vi "Display.vi"(0 "Data In":T4 {"time" format="%<%H:%M:%S%2u>T"}, 2 "Display State In":T2, 3 "Container State":T3) -> (6 "Data Out":T4 {"time" format="%<%H:%M:%S%2u>T"}, 7 "Display State Out":T2, 8 "Action":T1)   [LabVIEW 2015, in "Configurable Buffer.xctl"]
uses:
  Configurable Buffer.xctl
  Data.ctl
  <vilib>/_xctls/Container State.ctl
  State.ctl
  <vilib>/_xctls/Action.ctl
  <vilib>/_xctls/XControlSupport.lvlib
panel:
  out "plot":cluster{"Time":timestamp[], dbl[]}[](graph)
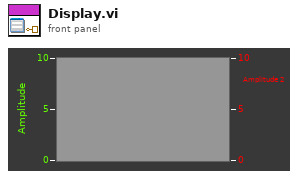
[diagram p1: front panel]
types:
  T1 = typedef "XControlSupport.lvlib/Action.ctl" = cluster{"Data Changed?":bool, "State Changed?":bool, "Action Name":string}
  T2 = typedef "Configurable Buffer.xctl/State.ctl" = cluster{"Plot Ref":refnum<vi>, "History":i32}
  T3 = typedef "XControlSupport.lvlib/Container State.ctl" = cluster{"Indicator?":bool, "Run Mode?":bool, " Refnum":refnum<vi>}
  T4 = typedef "Configurable Buffer.xctl/Data.ctl" = cluster{"Val":dbl[], "time":timestamp}
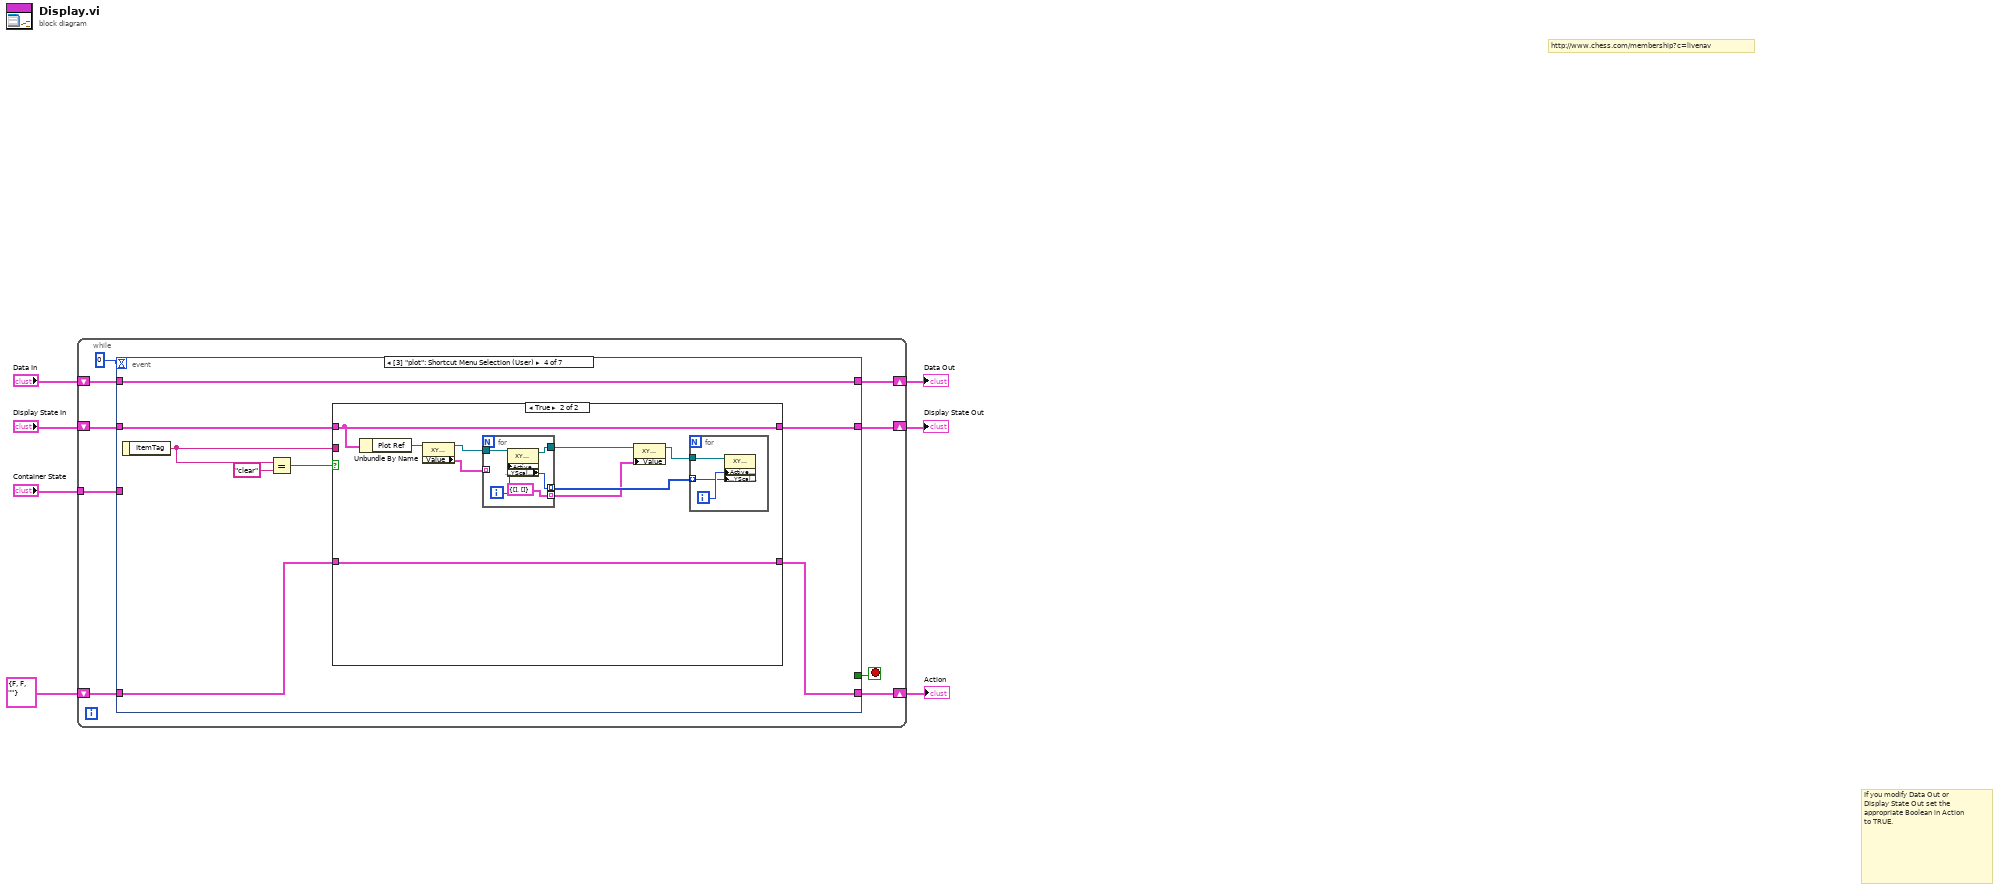
[diagram p0: block diagram]
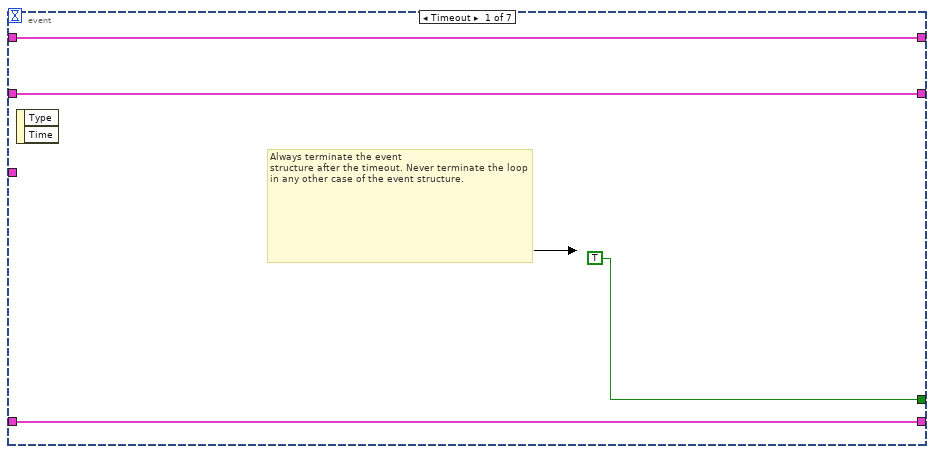
[diagram p2: hidden frame]
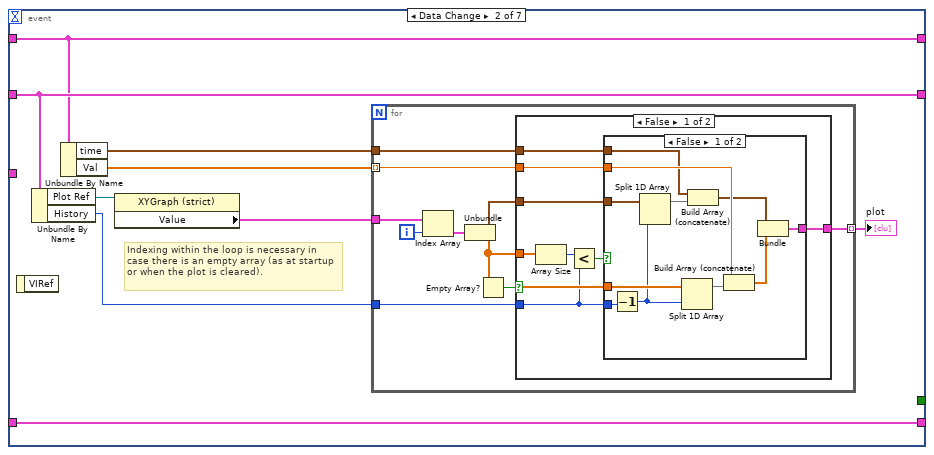
[diagram p3: hidden frame]
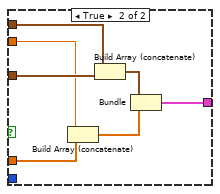
[diagram p4: hidden frame]
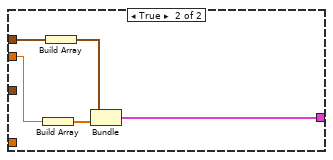
[diagram p5: hidden frame]
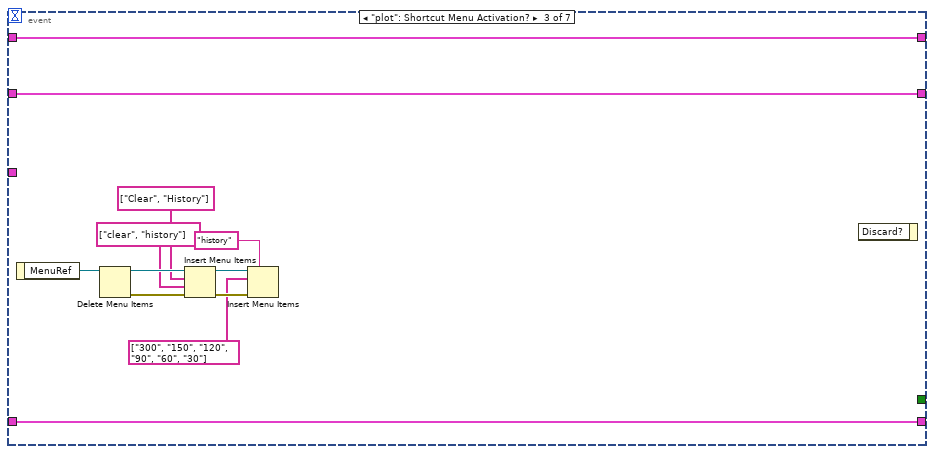
[diagram p6: hidden frame]
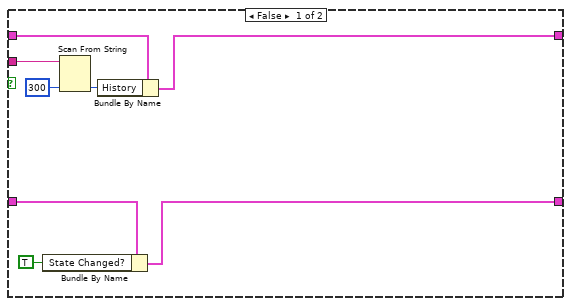
[diagram p7: hidden frame]
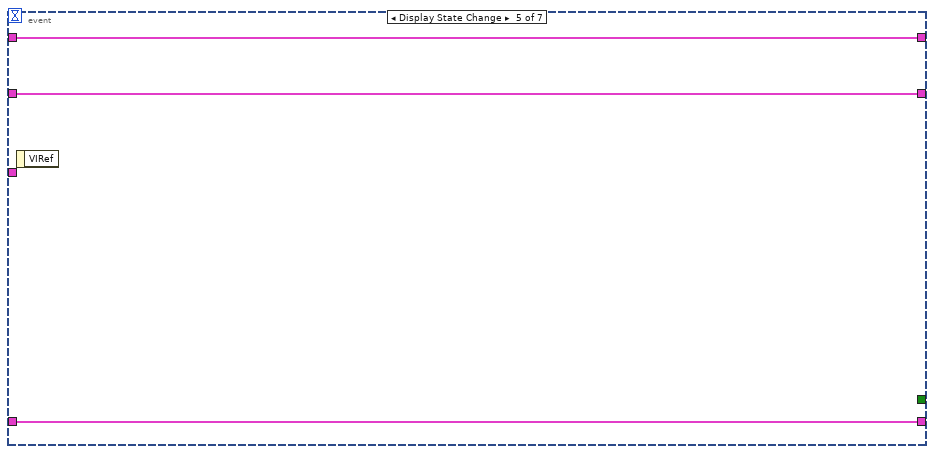
[diagram p8: hidden frame]
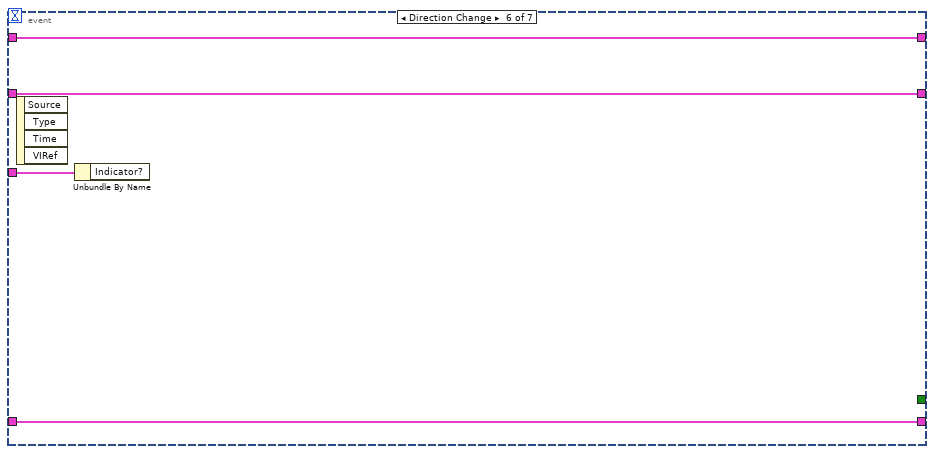
[diagram p9: hidden frame]
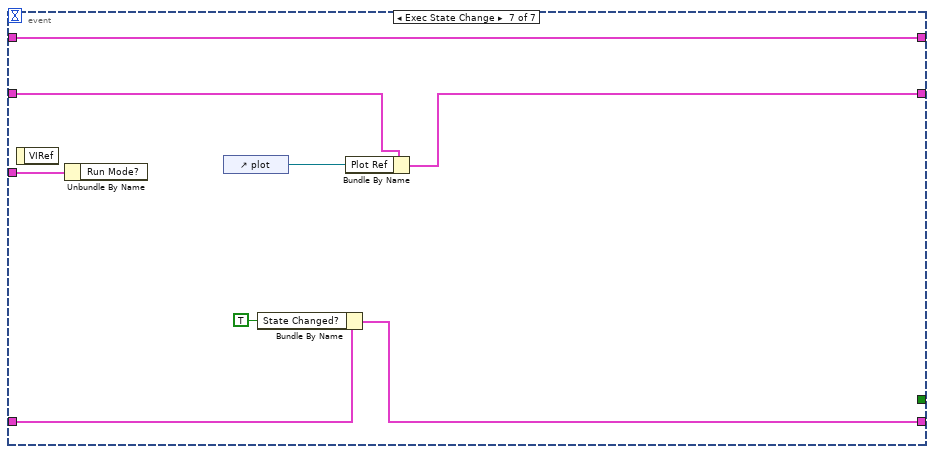
[diagram p10: hidden frame]
diagram:
  # "http://www.chess.com/membership?c=livenav"
  # "If you modify Data Out or\nDisplay State Out set the\nappropriate Boolean in Action\nto TRUE."
  n1 = while {
    shift-right: [w15] -> w4
    shift-left: "Display State In" -> [w16]
    tunnel: "Container State" -> [w12]
    shift-right: [w10] -> w7
    shift-left: "Data In" -> [w11]
    shift-right: [w8] -> w2
    shift-left: T1 {"Data Changed?"=FALSE, "State Changed?"=FALSE, "Action Name"=""} ("Action") -> [w9]
    stop <- w14 stop-if-true
    n2 = event shown="[3] \"plot\": Shortcut Menu Selection (User)" {
      selector: _ -> [_ _ _ _ _ _ _]
      dyn-events: _ -> [_ _ _ _ _ _ _]
      timeout: 0 -> [_ _ _ _ _ _ _]
      tunnel: w16 -> [w18 w29 w82 w86 w118 w121 w128]
      tunnel: [w18 w29 w82 w85 w118 w121 w127] -> w15
      tunnel: [TRUE _ _ _ _ _ _] -> w14
      tunnel: w12 -> [_ _ _ _ _ w122 w130]
      tunnel: w11 -> [w17 w28 w81 w90 w117 w120 w129]
      tunnel: [w17 w28 w81 w90 w117 w120 w129] -> w10
      tunnel: [w19 w27 w80 w83 w116 w119 w125] -> w8
      tunnel: w9 -> [w19 w27 w80 w84 w116 w119 w126]
      event Timeout {
        # "Always terminate the event\nstructure after the timeout. Never terminate the loop in any other case of the event structure."
        n3 = event-data() -> ()  [unwired: 1 in, 2 out]
      }
      event Data Change {
        # "Indexing within the loop is necessary in case there is an empty array (as at startup or when the plot is cleared)."
        n4 = event-data() -> ()  [unwired: 1 in, 1 out]
        n5 = Unbundle By Name(w29) -> ("Plot Ref"=w26:refnum<vi>, "History"=w21:i32)
        n6 = Unbundle By Name(w28) -> ("time"=w24:timestamp, "Val"=w23:dbl[])
        n7 = property on="Property Node" class="XYGraph (strict)"(reference=w26) -> ("Value"=w25:cluster{"Time":timestamp[], dbl[]}[])  [unwired: 1 in, 2 out]
        n8 = for {
          tunnel: w25 -> [w33]
          tunnel: w24 -> [w38]
          tunnel: w23 -> [w37] mode=indexing
          tunnel: [w36] -> w22 mode=indexing
          tunnel: w21 -> [w30]
          i -> [w31]
          n9 = Index Array(array=w33, index=w31) -> (element=w32:cluster{"Time":timestamp[], dbl[]})
          n10 = Unbundle(w32) -> ("Time"=w39:timestamp[], w35:dbl[])
          n11 = Empty Array?(array=w35) -> (empty?=w34:bool)
          n12 = case shown="False" w34 {
            tunnel: w39 -> [w45 _]
            tunnel: w38 -> [w44 w70]
            tunnel: w37 -> [w43 w69]
            tunnel: [w42 w66] -> w36
            tunnel: w35 -> [w41 _]
            tunnel: w30 -> [w40 _]
            frame False {
              n13 = Array Size(array=w41) -> (size(s)=w47:i32)
              n14 = Less?(x=w47, y=w40) -> (x < y?=w46:bool)
              n15 = case shown="False" w46 {
                tunnel: w41 -> [w57 w63]
                tunnel: w45 -> [w58 w64]
                tunnel: w44 -> [w53 w65]
                tunnel: w43 -> [w55 w62]
                tunnel: [w50 w59] -> w42
                tunnel: w40 -> [w49 _]
                frame False {
                  n16 = Decrement(x=w49) -> (x-1=w48:i32)
                  n17 = Split 1D Array(array=w58, index=w48) -> (first subarray=w54:timestamp[])  [unwired: 1 out]
                  n18 = Split 1D Array(array=w57, index=w48) -> (first subarray=w56:dbl[])  [unwired: 1 out]
                  n19 = Build Array (concatenate)(w53, w54) -> (w52:timestamp[])
                  n20 = Build Array (concatenate)(w55, w56) -> (w51:dbl[])
                  n21 = Bundle(w52, w51) -> (w50:cluster{timestamp[], dbl[]})  [unwired: 1 in]
                }
                frame True {
                  n22 = Build Array (concatenate)(w62, w63) -> (w60:dbl[])
                  n23 = Build Array (concatenate)(w65, w64) -> (w61:timestamp[])
                  n24 = Bundle(w61, w60) -> (w59:cluster{timestamp[], dbl[]})  [unwired: 1 in]
                }
              }
            }
            frame True {
              n25 = Build Array(w69) -> (w67:dbl[])
              n26 = Build Array(w70) -> (w68:timestamp[])
              n27 = Bundle(w68, w67) -> (w66:cluster{timestamp[], dbl[]})  [unwired: 1 in]
            }
          }
        }
        "plot" <- w22
      }
      event "plot": Shortcut Menu Activation? {
        n28 = event-data() -> ("MenuRef"=w79:refnum<k9>)  [unwired: 1 in]
        n29 = Delete Menu Items(9:w79) -> (0:w77:errorcluster, 3:w78:refnum<k9>)  [unwired: 3 in]
        n30 = Insert Menu Items(6:w77, 7:string[] ["clear", "history"] ("item tags"), 8:string[] ["Clear", "History"] ("item names"), 9:w78) -> (0:w73:errorcluster, 3:w74:refnum<k9>)  [unwired: 2 in, 1 out]
        n31 = Insert Menu Items(5:"history" ("menu tag"), 6:w73, 8:string[] ["300", "150", "120", "90", "60", "30"] ("item names"), 9:w74) -> ()  [unwired: 2 in, 3 out]
        n32 = event-data() -> ()  [unwired: 2 in, 1 out]
      }
      event "plot": Shortcut Menu Selection (User) {
        n33 = event-data() -> ("ItemTag"=w87:string)  [unwired: 1 in]
        n34 = Equal?(x=w87, y="clear") -> (x = y?=w88:bool)
        n35 = case shown="True" w88 {
          tunnel: w86 -> [w96 w107]
          tunnel: [w94 w107] -> w85
          tunnel: w87 -> [w98 _]
          tunnel: w84 -> [w93 w106]
          tunnel: [w91 w106] -> w83
          frame False {
            n36 = Bundle By Name(cluster=w93, "State Changed?"=TRUE) -> (w91:T1)
            n37 = Scan From String(input string=w98, default 1=300) -> (output 1=w95:i32)  [unwired: 3 in, 3 out]
            n38 = Bundle By Name(cluster=w96, "History"=w95) -> (w94:T2)
          }
          frame True {
            n39 = Unbundle By Name(w107) -> ("Plot Ref"=w105:refnum<vi>)
            n40 = property class="XYGraph (strict)"(reference=w105) -> (reference out=w103:refnum<vi>, "Value"=w104:cluster{"Time":timestamp[], dbl[]}[])  [unwired: 1 in, 1 out]
            n41 = for {
              tunnel: w104 -> [_] mode=indexing
              tunnel: w103 -> [w115]
              tunnel: [w113] -> w100 mode=indexing
              tunnel: [w112] -> w102
              tunnel: [cluster{"Time":timestamp[], dbl[]} {"Time"=[], []}] -> w99 mode=indexing
              i -> [w114]
              n42 = property class="XYGraph (strict)"(reference=w115, "Active Plot"=w114) -> (reference out=w112:refnum<vi>, "Plot.YScaleIdx"=w113:u32)  [unwired: 1 in, 1 out]
            }
            n43 = property class="XYGraph (strict)"(reference=w102, "Value"=w99) -> (reference out=w101:refnum<vi>)  [unwired: 1 in, 1 out]
            n44 = for {
              tunnel: w101 -> [w109]
              tunnel: w100 -> [w108] mode=indexing
              i -> [w110]
              n45 = property class="XYGraph (strict)"(reference=w109, "Active Plot"=w110, "Plot.YScaleIdx"=w108) -> ()  [unwired: 1 in, 2 out]
            }
          }
        }
      }
      event Display State Change {
        n46 = event-data() -> ()  [unwired: 1 in, 1 out]
      }
      event Direction Change {
        n47 = event-data() -> ()  [unwired: 1 in, 4 out]
        n48 = Unbundle By Name(w122) -> ()  [unwired: 1 out]
      }
      event Exec State Change {
        n49 = event-data() -> ()  [unwired: 1 in, 1 out]
        n50 = Unbundle By Name(w130) -> ()  [unwired: 1 out]
        n51 = control-ref of="plot"() -> (w123:refnum<vi>)
        n52 = Bundle By Name(cluster=w126, "State Changed?"=TRUE) -> (w125:T1)
        n53 = Bundle By Name(cluster=w128, "Plot Ref"=w123) -> (w127:T2)
      }
    }
  }
  "Display State Out" <- w4
  "Data Out" <- w7
  "Action" <- w2
